vi "Send Direct Command.vi"(0 "VISA resource name":refnum<visa-resource-name>, 1 "Select Action":u16(ring) items=["Ping", "Read", "Write", "Registered Write", "Action", "Reset", "Sync Write"], 2 "Motor ID (0)":u8, 3 "Address":u8, 4 "Parameters":string, 5 "Error in (no error)":errorcluster) -> (14 "VISA resource name out":refnum<visa-resource-name>, 17 "Command to Serial":string, 19 "Error out":errorcluster)   [LabVIEW 2016, in "Dynamixel Motor.lvlib"]
doc: "Using any of the six basic commands for the Dynamixel motor, this VI allows you to send any set of parameters to the motor(s). This is a Low-Level VI that is used by other VIs."
uses:
  Dynamixel Motor.lvlib
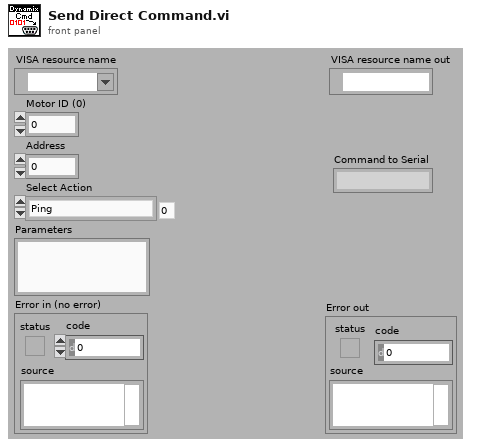
[diagram p1: front panel]
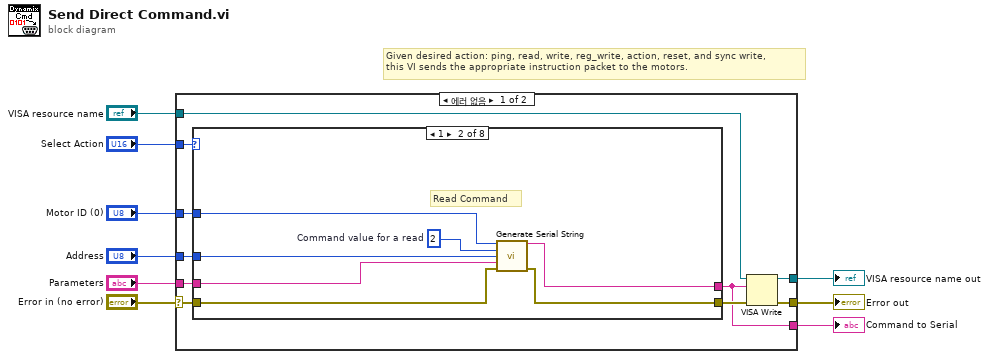
[diagram p0: block diagram]
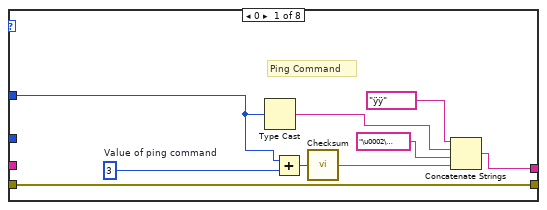
[diagram p2: hidden frame]
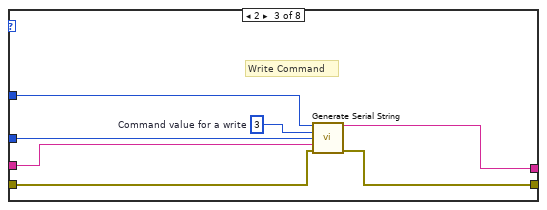
[diagram p3: hidden frame]
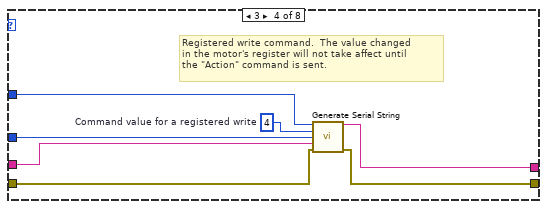
[diagram p4: hidden frame]
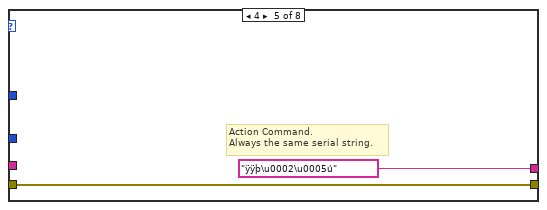
[diagram p5: hidden frame]
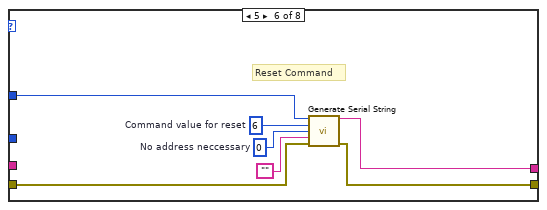
[diagram p6: hidden frame]
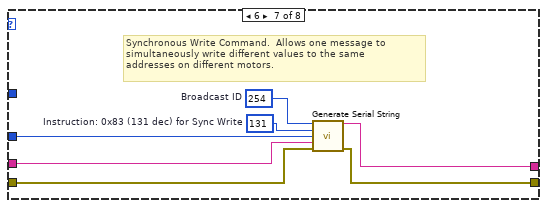
[diagram p7: hidden frame]
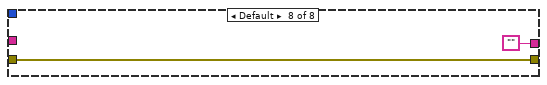
[diagram p8: hidden frame]
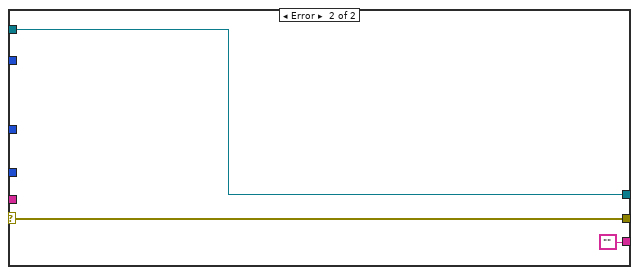
[diagram p9: hidden frame]
diagram:
  # "Given desired action: ping, read, write, reg_write, action, reset, and sync write,\nthis VI sends the appropriate instruction packet to the motors."
  n1 = case shown="에러 없음" "Error in (no error)" {
    selector: "Error in (no error)" -> [w15 w70]
    tunnel: "Parameters" -> [w19 _]
    tunnel: "Address" -> [w18 _]
    tunnel: "Motor ID (0)" -> [w17 _]
    tunnel: "Select Action" -> [w16 _]
    tunnel: [w12 w70] -> w6
    tunnel: [w14 w69] -> w5
    tunnel: "VISA resource name" -> [w11 w69]
    tunnel: [w10 ""] -> w1
    frame No Error {
      n2 = case shown="1" w16 {
        tunnel: w15 -> [w20 w31 w38 w44 w50 w53 w61 w66]
        tunnel: [w20 w29 w37 w43 w50 w52 w60 w66] -> w13
        tunnel: w17 -> [w23 w35 w42 w49 _ w58 _ _]
        tunnel: w18 -> [_ w34 w41 w48 _ _ w65 _]
        tunnel: w19 -> [_ w32 w40 w47 _ _ w64 _]
        tunnel: [w21 w30 w36 w45 "ÿÿþ\u0002\u0005ú" w54 w62 ""] -> w10
        frame 0 {
          w26 = u8 3  # Value of ping command
          # "Ping Command"
          n3 = Type Cast(x=w23) -> (*(type *) &x=w22:string)  [unwired: 1 in]
          n4 = Add(x=w23, y=w26) -> (x+y=w25:u8)
          n5 = call "Checksum.vi"("Sum of bytes"=w25) -> ("Checksum String"=w24:string)
          n6 = Concatenate Strings("ÿÿ", w22, "\u0002\u0001", w24) -> (w21:string)
        }
        frame 1 {
          w33 = u8 2  # Command value for a read
          # "Read Command"
          n7 = call "Generate Serial String.vi"("Motor ID"=w35, "Command"=w33, "Address"=w34, "Parameters"=w32, "Error in (no error)"=w31) -> ("Command to Serial"=w30:string, "error out"=w29:errorcluster)  [unwired: 9 in]
        }
        frame 2 {
          w39 = u8 3  # Command value for a write
          # "Write Command"
          n8 = call "Generate Serial String.vi"("Motor ID"=w42, "Command"=w39, "Address"=w41, "Parameters"=w40, "Error in (no error)"=w38) -> ("Command to Serial"=w36:string, "error out"=w37:errorcluster)  [unwired: 9 in]
        }
        frame 3 {
          w46 = u8 4  # Command value for a registered write
          # "Registered write command.  The value changed \nin the motor's register will not take affect until \nthe \"Action\" command is sent."
          n9 = call "Generate Serial String.vi"("Motor ID"=w49, "Command"=w46, "Address"=w48, "Parameters"=w47, "Error in (no error)"=w44) -> ("Command to Serial"=w45:string, "error out"=w43:errorcluster)  [unwired: 9 in]
        }
        frame 4 {
          # "Action Command.\nAlways the same serial string."
        }
        frame 5 {
          w55 = u8 0  # No address neccessary
          w56 = u8 6  # Command value for reset
          # "Reset Command"
          n10 = call "Generate Serial String.vi"("Motor ID"=w58, "Command"=w56, "Address"=w55, "Parameters"="", "Error in (no error)"=w53) -> ("Command to Serial"=w54:string, "error out"=w52:errorcluster)  [unwired: 9 in]
        }
        frame 6 {
          w59 = u8 254  # Broadcast ID
          w63 = u8 131  # Instruction: 0x83 (131 dec) for Sync Write
          # "Synchronous Write Command.  Allows one message to\nsimultaneously write different values to the same \naddresses on different motors."
          n11 = call "Generate Serial String.vi"("Motor ID"=w59, "Command"=w63, "Address"=w65, "Parameters"=w64, "Error in (no error)"=w61) -> ("Command to Serial"=w62:string, "error out"=w60:errorcluster)  [unwired: 9 in]
        }
        frame Default {
        }
      }
      n12 = VISA Write(VISA resource name=w11, write buffer=w10, error in (no error)=w13) -> (VISA resource name out=w14:refnum<visa-resource-name>, error out=w12:errorcluster)  [unwired: 1 out]
    }
    frame Error {
    }
  }
  "Error out" <- w6
  "VISA resource name out" <- w5
  "Command to Serial" <- w1
